vi "write state.vi"(8 "error in (no error)":errorcluster, 10 "state":string, 11 "Channel in":refnum<class "Channel.lvclass">) -> (0 "error out":errorcluster, 3 "Channel out":refnum<class "Channel.lvclass">)   [LabVIEW 2018, in "Channel.lvclass"]
uses:
  Channel.lvclass
  Channel.lvclass/Channel.ctl
  State Machine/CCS_State Machine.lvclass
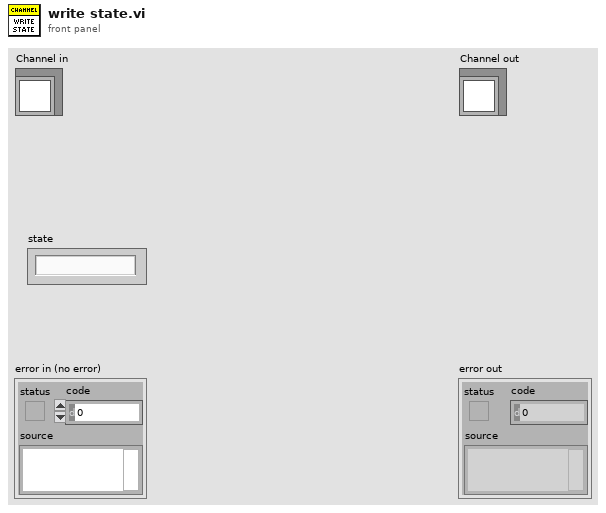
[diagram p1: front panel]
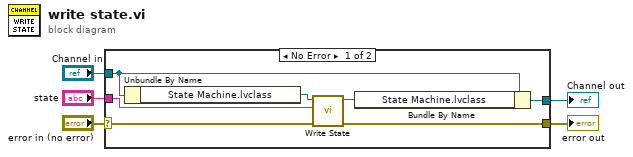
[diagram p0: block diagram]
diagram:
  n1 = case shown="No Error" "error in (no error)" {
    selector: "error in (no error)" -> [w8 w14]
    tunnel: [w7 w14] -> w4
    tunnel: [w9 w13] -> w2
    tunnel: "Channel in" -> [w10 w13]
    tunnel: "state" -> [w6 _]
    frame No Error {
      n2 = Unbundle By Name(w10) -> ("State Machine.lvclass"=w11:refnum<class "CCS_State Machine.lvclass">)
      n3 = call-dynamic "Write State.vi"("error in (no error)"=w8, "State"=w6, "State Machine in"=w11) -> ("error out"=w7:errorcluster, "State Machine out"=w12:refnum<class "CCS_State Machine.lvclass">)  [unwired: 7 in]
      n4 = Bundle By Name(cluster=w10, "State Machine.lvclass"=w12) -> (w9:refnum<class "Channel.lvclass">)
    }
    frame Error {
    }
  }
  "error out" <- w4
  "Channel out" <- w2
